vi "SSL_Connect.vi"(8 "error in (no error)":errorcluster, 11 "SSL in":refnum<class "SSL.lvclass">) -> (0 "error out":errorcluster, 3 "SSL out":refnum<class "SSL.lvclass">)   [LabVIEW 2013, in "OpenSSL Socket.lvlib" / "SSL.lvclass"]
uses:
  SSL.lvclass
  SSL-Lib/SSL-Lib.lvclass/SSL-Lib.ctl
  SSL.lvclass/SSL.ctl
  SSL-Lib/Read SSL Library Path.vi
  Read Handle.vi
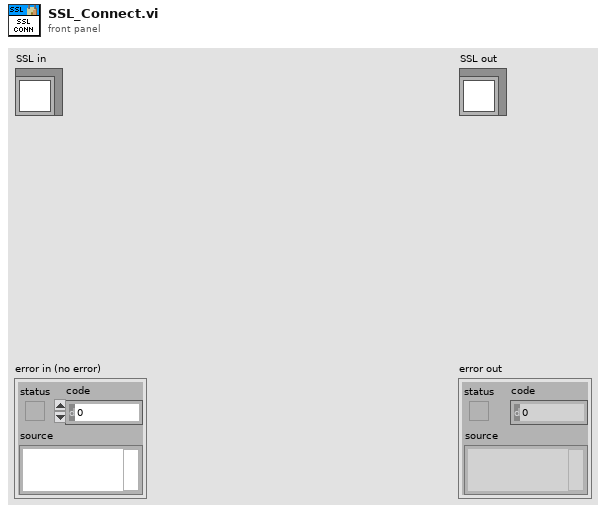
[diagram p1: front panel]
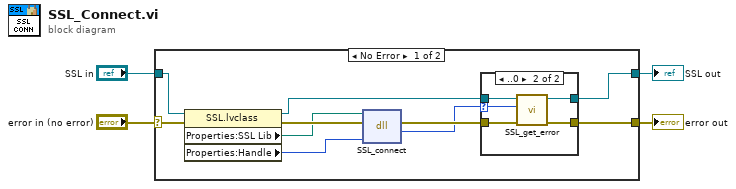
[diagram p0: block diagram]
diagram:
  n1 = case shown="No Error" "error in (no error)" {
    selector: "error in (no error)" -> [w14 w23]
    tunnel: [w8 w23] -> w3
    tunnel: [w6 w22] -> w1
    tunnel: "SSL in" -> [w12 w22]
    frame No Error {
      n2 = property class="SSL.lvclass"(reference=w12, error in=w14) -> (reference out=w7:refnum<class "SSL.lvclass">, error out=w13:errorcluster, "Properties:SSL Lib"=w11:path, "Properties:Handle"=w10:u64)
      n3 = dll-call lib="C:/Program Files (x86)/National Instruments/Shared/nissl/NIssleay32.dll" fn="SSL_connect"(path in=w11, error in=w13, "*SSL"=w10) -> (error out=w9:errorcluster, "return"=w5:i32)  [unwired: 2 in, 1 out]
      n4 = case shown="..0" w5 {
        selector: w5 -> [_ w17]
        tunnel: w9 -> [w15 w21]
        tunnel: [w15 w20] -> w8
        tunnel: w7 -> [w16 w19]
        tunnel: [w16 w18] -> w6
        frame Default {
        }
        frame ..0 {
          n5 = call "SSL_get_error.vi"("error in (no error)"=w21, "SSL return code"=w17, "SSL-Lib in"=w19) -> ("error out"=w20:errorcluster, "SSL-Lib out"=w18:refnum<class "SSL.lvclass">)  [unwired: 6 in, 1 out]
        }
      }
    }
    frame Error {
    }
  }
  "error out" <- w3
  "SSL out" <- w1
